vi "WS1050_36 DUT SData Ver1.5a.vi"(0 "TMN DC\\CAP Data Log File Path":path=path "C:/temp", 1 "Lot#":string="WS1050", 2 "Total Delta C1(pF)":string[](array[string]), 3 "VSA_V1":string[][](array[string]), 4 "Wafer#":string="T7", 5 "File Name":string="Test Data", 6 "Total Delta C2(pF)":string[](array[string]), 7 "error in":errorcluster, 8 "TP/Comment":T1={"Test Program"="Multi Socket", "Comment"="HD_Cycling", "DVA"="", "EFUSE CAL"="", "CP HD/CYC"="", "VDD"="", "Duty Cycle"="", "V_Test(V)"="", "V_VPI(V)"="", "Freq(Hz)"="", "Board#"=""}, 9 "EFuse":string[](array[string])=["NC", "NC", "NC", "NC", "NC", "NC", "NC", "NC", "NC", "NC", "NC", "NC", "NC", "NC", "NC", "NC", "NC", "NC", "NC", "NC", "NC", "NC", "NC", "NC", "NC", "NC", "NC", "NC", "NC", "NC", "NC", "NC", "NC", "NC", "NC", "NC"], 10 "Data Output C3":string[][](table), 11 "Temperature":string="WS1033", 12 "VSA_V2":string[][](array[string]), 13 "VPI C3":string[][](array[string]), 14 "Data Output C1":string[][](table), 15 "VPI C2":string[][](array[string]), 16 "SN":string[](array[string])=["1", "2", "3", "4", "5", "6", "7", "8", "9", "10", "11", "12", "13", "14", "15", "16", "17", "18", "19", "20", "21", "22", "23", "24", "25", "26", "27", "28", "29", "30", "31", "32", "33", "34", "35", "36"], 17 "R/W Status":string[](array[string])=["PASS", "PASS", "PASS", "PASS", "PASS", "PASS", "PASS", "PASS", "PASS", "PASS", "PASS", "PASS", "PASS", "PASS", "PASS", "PASS", "PASS", "PASS", "PASS", "PASS", "PASS", "PASS", "PASS", "PASS", "PASS", "PASS", "PASS", "PASS", "PASS", "PASS", "PASS", "PASS", "PASS", "PASS", "PASS", "PASS"], 18 "Cap Header":string[](array[string]), 20 "HD/Cycles Completed":string="Test Data", 21 "Data Output C2":string[][](table), 22 "STress Beams":string="STD", 23 "VSA_V3":string[][](array[string]), 24 "Current":string[](array[string]), 25 "VPI C1":string[][](array[string]), 26 "Total Delta C3(pF)":string[](array[string])) -> (27 "error out":errorcluster)   [LabVIEW 2012]
panel:
  in  "Bin":string[](array[string])=["NC", "NC", "NC", "NC", "NC", "NC", "NC", "NC", "NC", "NC", "NC", "NC", "NC", "NC", "NC", "NC", "NC", "NC", "NC", "NC", "NC", "NC", "NC", "NC", "NC", "NC", "NC", "NC", "NC", "NC", "NC", "NC", "NC", "NC", "NC", "NC"]
  # "*********** Do Not Remove ***********\nCompany:  WiSpry Inc\n20 Fairbanks Ste 198 Irvine CA 92618\n\nAuthor:  Andy V Tran\nCreated:  09/17/2014\nLabVIEW 2012 Suite\nTP:  Multi-Socket Save Data ver1.0\n*****************************************"
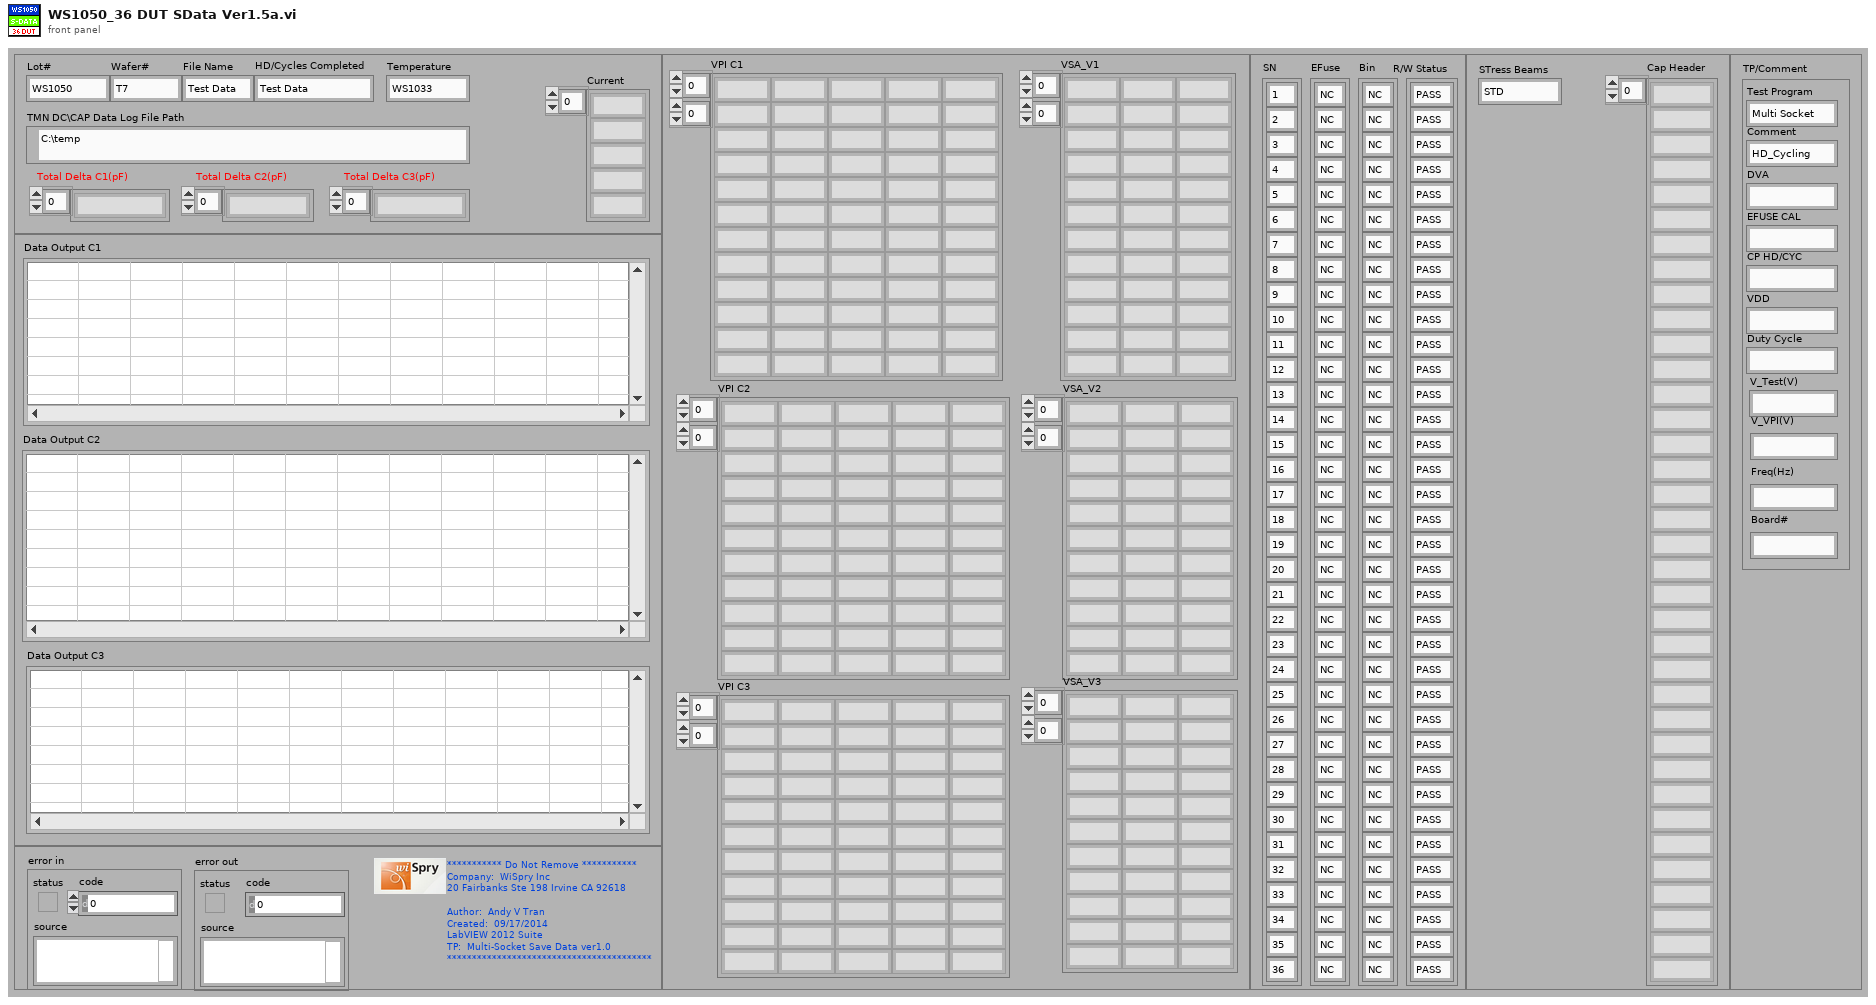
[diagram p1: front panel]
types:
  T1 = cluster{"Test Program":string, "Comment":string, "DVA":string, "EFUSE CAL":string, "CP HD/CYC":string, "VDD":string, "Duty Cycle":string, "V_Test(V)":string, "V_VPI(V)":string, "Freq(Hz)":string, "Board#":string}
  T2 = enum16{"open", "replace", "create", "open or create", "replace or create", "replace or create with confirmation"}
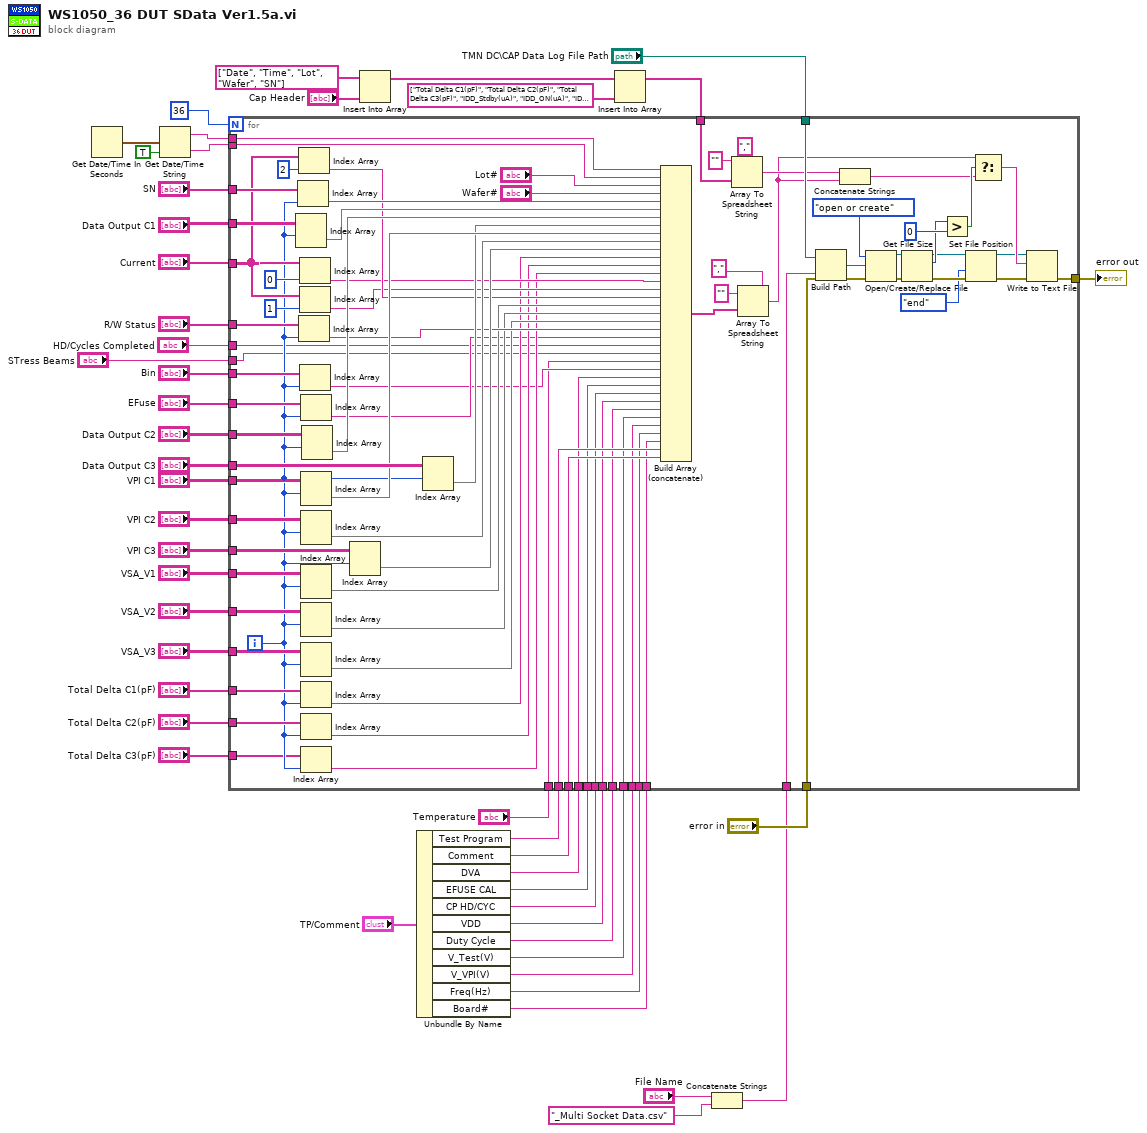
[diagram p0: block diagram]
diagram:
  n1 = Get Date/Time In Seconds() -> (seconds since 1Jan1904=w27:timestamp)
  n2 = Get Date/Time String(seconds (now)=w27, want seconds? (F)=TRUE) -> (date string=w35:string, time string=w36:string)  [unwired: 1 in]
  n3 = Insert Into Array(array=string[] ["Date", "Time", "Lot", "Wafer", "SN"], new element="Cap Header") -> (w13:string[])  [unwired: 1 in]
  n4 = Unbundle By Name("TP/Comment") -> ("Test Program"=w40:string, "Comment"=w39:string, "DVA"=w12:string, "EFUSE CAL"=w11:string, "CP HD/CYC"=w10:string, "VDD"=w9:string, "Duty Cycle"=w8:string, "V_Test(V)"=w7:string, "V_VPI(V)"=w6:string, "Freq(Hz)"=w4:string, "Board#"=w3:string)
  n5 = Insert Into Array(array=w13, new element=string[] ["Total Delta C1(pF)", "Total Delta C2(pF)", "Total Delta C3(pF)", "IDD_Stdby(uA)", "IDD_ON(uA)", "IDD_OFF(uA)", "VSA_V1_(V)", "VSA_V1_C1(pF)", "VSA_V1_C2(pF)", "VSA_V1_C3(pF)", "VSA_V2(V)", "VSA_V2_C1(pF)", "VSA_V2_C2(pF)", "VSA_V2_C3(pF)", "VSA_V3(V)", "VSA_V3_C1(pF)", "VSA_V3_C2(pF)", "VSA_V3_C3(pF)", "R/W Status(P/F)", "EFuse RB", "HD-CYC Completed", "Stress Beams", "Temperature", "Bin", "DVA ON/OFF", "CAL ON/OFF", "CP_HD/CYC", "VDD", "Duty Cycle(%)", "V_Test(V)", "V_VPI(V)", "Freq(Hz)", "Board", "Test Program", "Comment"]) -> (w17:string[])  [unwired: 1 in]
  n6 = Concatenate Strings("File Name", "_Multi Socket Data.csv" ("string")) -> (w43:string)
  n7 = for {
    N: 36 -> [_]
    tunnel: "TMN DC\\CAP Data Log File Path" -> [w132]
    tunnel: w17 -> [w131]
    tunnel: "error in" -> [w92]
    tunnel: w43 -> [w130]
    tunnel: [w108] -> w42
    tunnel: "SN" -> [w107]
    tunnel: "Current" -> [w99]
    tunnel: w40 -> [w61]
    tunnel: w39 -> [w62]
    tunnel: "Bin" -> [w106]
    tunnel: "R/W Status" -> [w105]
    tunnel: w36 -> [w82]
    tunnel: w35 -> [w81]
    tunnel: "Data Output C1" -> [w104]
    tunnel: "Data Output C2" -> [w103]
    tunnel: "VPI C1" -> [w98]
    tunnel: "VPI C2" -> [w97]
    tunnel: "EFuse" -> [w96]
    tunnel: "VSA_V1" -> [w95]
    tunnel: "VSA_V2" -> [w94]
    tunnel: "VSA_V3" -> [w93]
    tunnel: "VPI C3" -> [w91]
    tunnel: "Data Output C3" -> [w90]
    tunnel: "Total Delta C1(pF)" -> [w80]
    tunnel: "Total Delta C2(pF)" -> [w79]
    tunnel: "Total Delta C3(pF)" -> [w77]
    tunnel: w12 -> [w52]
    tunnel: w11 -> [w53]
    tunnel: w10 -> [w54]
    tunnel: w9 -> [w55]
    tunnel: w8 -> [w56]
    tunnel: w7 -> [w57]
    tunnel: w6 -> [w58]
    tunnel: "HD/Cycles Completed" -> [w63]
    tunnel: w4 -> [w59]
    tunnel: w3 -> [w60]
    tunnel: "Temperature" -> [w50]
    tunnel: "STress Beams" -> [w49]
    i -> [w78]
    n8 = Index Array(array=w104, index (row)=w78) -> (element=w84:string[])  [unwired: 1 in]
    n9 = Index Array(array=w107, index=w78) -> (element=w83:string)
    n10 = Index Array(array=w99, index=2) -> (element=w72:string)
    n11 = Index Array(array=w105, index=w78) -> (element=w76:string)
    n12 = Index Array(array=w99, index=0) -> (element=w70:string)
    n13 = Index Array(array=w99, index=1) -> (element=w71:string)
    n14 = Index Array(array=w106, index=w78) -> (element=w51:string)
    n15 = Index Array(array=w96, index=w78) -> (element=w64:string)
    n16 = Index Array(array=w98, index (row)=w78) -> (element=w87:string[])  [unwired: 1 in]
    n17 = Index Array(array=w97, index (row)=w78) -> (element=w88:string[])  [unwired: 1 in]
    n18 = Index Array(array=w95, index (row)=w78) -> (element=w73:string[])  [unwired: 1 in]
    n19 = Index Array(array=w94, index (row)=w78) -> (element=w74:string[])  [unwired: 1 in]
    n20 = Index Array(array=w93, index (row)=w78) -> (element=w75:string[])  [unwired: 1 in]
    n21 = Index Array(array=w80, index=w78) -> (element=w69:string)
    n22 = Index Array(array=w79, index=w78) -> (element=w68:string)
    n23 = Index Array(array=w77, index=w78) -> (element=w67:string)
    n24 = Index Array(array=w103, index (row)=w78) -> (element=w85:string[])  [unwired: 1 in]
    n25 = Index Array(array=w91, index (row)=w78) -> (element=w89:string[])  [unwired: 1 in]
    n26 = Index Array(array=w90, index (row)=w78) -> (element=w86:string[])  [unwired: 1 in]
    n27 = Build Array (concatenate)(w81, w82, "Lot#", "Wafer#", w83, w84, w85, w86, w87, w88, w89, w69, w68, w67, w70, w71, w72, w73, w74, w75, w76, w64, w63, w49, w50, w51, w52, w53, w54, w55, w56, w57, w58, w59, w60, w61, w62) -> (w109:string[])
    n28 = Array To Spreadsheet String(delimiter (Tab)=",", array=w131, 3:"" ("format string")) -> (spreadsheet string=w112:string)
    n29 = Array To Spreadsheet String(delimiter (Tab)=",", array=w109, 3:"" ("format string")) -> (spreadsheet string=w110:string)
    n30 = Build Path(base path=w132, name or relative path=w130) -> (appended path=w124:path)
    n31 = Concatenate Strings(w112, w110) -> (w111:string)
    n32 = Open/Create/Replace File(file path (use dialog)=w124, error in=w92, operation (0:open)=T2."open or create") -> (refnum out=w122:refnum<file>, error out=w125:errorcluster)  [unwired: 4 out]
    n33 = Get File Size(file=w122, error in=w125) -> (refnum out=w117:refnum<file>, size (in bytes)=w121:i64, 0:w119:errorcluster)
    n34 = Greater?(x=w121, y=i64 0) -> (0:w126:bool)
    n35 = Set File Position(refnum=w117, from (0:start)=enum16{"start", "end", "current"}."end", error in=w119) -> (refnum out=w116:refnum<file>, error out=w118:errorcluster)  [unwired: 1 out]
    n36 = Select(t=w110, s=w126, f=w111) -> (s? t:f=w123:string)
    n37 = Write to Text File(file (use dialog)=w116, text=w123, error in=w118) -> (error out=w108:errorcluster)  [unwired: 3 out]
  }
  "error out" <- w42
